vi "HFRR ADV v01.vi"() -> ()   [LabVIEW 2025] (continued)
          tunnel: w2263 -> [w2288 w2293]
          tunnel: [w2288 w2297] -> w2267
          tunnel: w2269 -> [w2287 w2292]
          tunnel: [w2287 w2295] -> w2275
          tunnel: w2265 -> [_ w2291]
          tunnel: [_ w2294] -> _
          frame False {
            # "DATA  WRITE LOOP"
          }
          frame True {
            n1901 = Concatenate Strings(w2291, "\r\n") -> (w2290:string)
            n1902 = VISA Write(VISA resource name=w2293, write buffer=w2290, error in (no error)=w2292) -> (VISA resource name out=w2297:refnum<visa-resource-name>, return count=w2294:u32, error out=w2296:errorcluster)
            n1903 = flat-sequence {
              tunnel: w2296 -> [w2299]
              tunnel: [w2299] -> w2295
              frame #0 {
                n1904 = local write "Due Write"("" ("Command")) -> ()
                n1905 = Wait (ms)(milliseconds to wait=u32 5) -> ()  [unwired: 1 out]
              }
            }
          }
        }
        "Port 2a" <- TRUE ("Port 2a")
      }
      frame Error {
        w2316 = u16 0 items=["None", "XON/XOFF", "RTS/CTS", "XON/XOFF & RTS/CTS", "DTR/DSR", "XON/XOFF & DTR/DSR"] ("flow control (0:none)  2")
        w2314 = u16 10 items=["1.0"=10, "1.5"=15, "2.0"=20] ("stop bits 2")
        w2312 = u16 0 items=["None", "Odd", "Even", "Mark", "Space"] ("parity 2")
        w2313 = u32 10000  # timeout (10sec)
        n1906 = VISA Clear(VISA resource name=w2308, error in (no error)=w2305) -> (VISA resource name out=w2307:refnum<visa-resource-name>, error out=w2306:errorcluster)
        n1907 = VISA Close(VISA resource name=w2307, error in (no error)=w2306) -> (error out=w2309:errorcluster)
        n1908 = call <vilib>:"Clear Errors.vi"("error in (no error)"=w2309) -> ()  [unwired: 5 in, 2 out]
        n1909 = local write "Port 2a"(FALSE ("Port 2a")) -> ()
        n1910 = local read "Com Port 2"() -> (w2302:refnum<visa-resource-name>)
        "visa due" <- w2302
        n1911 = call-poly "VISA Configure Serial Port"("VISA resource name"=w2302, "timeout (10sec)"=w2313, "baud rate (9600)"=u32 250000 ("baud rate  2"), "data bits (8)"=u16 8 ("data bits  2"), "parity (0:none)"=w2312, "stop bits (10: 1 bit)"=w2314, "flow control (0:none)"=w2316) -> ("VISA resource name out"=w2317:refnum<visa-resource-name>, "error out"=w2318:errorcluster)  [unwired: 7 in]
        n1912 = flat-sequence {
          tunnel: w2317 -> [w2320]
          tunnel: w2318 -> [w2319]
          tunnel: [w2320] -> w2310
          tunnel: [w2319] -> w2303
          frame #0 {
            n1913 = Wait (ms)(milliseconds to wait=u32 50) -> ()  [unwired: 1 out]
          }
        }
        "Residual Due" <- ""
      }
    }
    "error out 9" <- w2244
    n1914 = local read "Quit"() -> (w2246:bool)
    "Error Due" <- w2251
  }
  n1915 = local write "FRICVALZ"(0.0 ("FRICVALZ")) -> ()
  n1916 = property on="RUN" class="Bool (strict)"("Visible"=TRUE) -> ()  [unwired: 2 in, 2 out]
  n1917 = while {
    tunnel: [w2335] -> _
    tunnel: [w2322] -> w59
    i -> [w2335]
    stop <- w2322 stop-if-true
    n1918 = local read "conststatus"() -> (w2326:dbl)
    n1919 = local read "Main Tab"() -> (w2324:T4)
    n1920 = local read "EDIT"() -> (w2341:bool)
    n1921 = local read "Rate"() -> (w2340:dbl)
    n1922 = case shown="True" w2341 {
      tunnel: [FALSE TRUE] -> _
      frame False {
      }
      frame True {
      }
    }
    n1923 = Equal?(x=w2324, y=T28."About" ("Main Tab")) -> (x = y?=w2333:bool)
    n1924 = Equal?(x=w2326, y=0.0) -> (x = y?=w2327:bool)
    n1925 = Divide(x=1.0, y=w2340) -> (x/y=w2336:dbl)
    "Time 2" <- w2336
    n1926 = case shown="True" w2327 {
      frame False {
      }
      frame True {
        # "C:\\WinDucom\\calibrate WO 2391.dcf"
        n1927 = local write "Lan flag"(22) -> ()
        n1928 = local write "conststatus"(10.0 ("rpm value : 2")) -> ()
        n1929 = String To Path(string="C:\\LAB-IQ\\calibrate WO 2472.dcf") -> (path=w2347:path)
        n1930 = Open/Create/Replace File "Open File"(file path (use dialog)=w2347) -> (refnum out=w2345:refnum<file>)  [unwired: 5 in, 2 out]
        n1931 = for {
          N: 23 -> [_]
          tunnel: w2345 -> [w2356]
          i -> [w2350]
          (unwired) TRUE ("line mode (F)")
          n1932 = Read from Text File "Read File"(file (use dialog)=w2356) -> (text=w2355:string)  [unwired: 3 in, 3 out]
          n1933 = Match Pattern(string=w2355, regular expression="]") -> (after substring=w2353:string)  [unwired: 1 in, 3 out]
          n1934 = String Subset(string=w2355, offset (0)=5, length (rest)=10 ("length (rest)")) -> (substring=w2348:string)
          n1935 = Fract/Exp String To Number(string=w2348) -> (number=w2349:dbl)  [unwired: 3 in, 1 out]
          n1936 = Match Pattern(string=w2353, regular expression="-") -> (before substring=w2351:string)  [unwired: 1 in, 3 out]
          n1937 = case shown="10" w2350 {
            tunnel: w2349 -> [_ _ _ _ _ _ _ _ _ _ w2363 _ _ _ _ _ _ _ _ _ _ _ _ _]
            tunnel: w2351 -> [_ _ _ _ w2359 w2360 w2361 _ _ _ _ _ _ _ _ _ _ _ _ _ w2364 w2365 w2366 _]
            frame 0 {
            }
            frame 1 {
            }
            frame 2 {
            }
            frame 3 {
            }
            frame 4 {
              n1938 = local write "Com Port 1"(w2359) -> ()
            }
            frame 5 {
              n1939 = local write "Com Port 2"(w2360) -> ()
              n1940 = local write "visa due"(w2360) -> ()
            }
            frame 6 {
              n1941 = String To Path(string=w2361) -> (path=w2362:path)
              n1942 = local write "File Path"(w2362) -> ()
              "String" <- w2361
            }
            frame 7 {
            }
            frame 8 {
            }
            frame 9 {
            }
            frame 10 {
              n1943 = local write "Language Selection"(w2363) -> ()
            }
            frame 11 {
            }
            frame 12 {
            }
            frame 13 {
            }
            frame 14 {
            }
            frame 15 {
            }
            frame 16 {
            }
            frame 17 {
            }
            frame 18 {
            }
            frame 21 {
            }
            frame 22 {
              n1944 = local write "Com Port 3"(w2364) -> ()
            }
            frame 20 {
              n1945 = local write "Camera Port :"(w2365) -> ()
            }
            frame 19 {
              n1946 = local write "C3 :"(w2366) -> ()
            }
            frame 23, Default {
            }
          }
        }
      }
    }
    n1947 = Select(t=u32 2500 ("milliseconds to wait"), s=w2333, f=u32 500 ("milliseconds to wait")) -> (s? t:f=w2331:u32)
    n1948 = Multiply(x=w2336, y=w2331) -> (x*y=w2338:dbl)
    n1949 = call "Elapsed Time2"("Time Target (s)"=w2338, "Auto Reset"=TRUE) -> ("Time has Elapsed"=w2328:bool)  [unwired: 10 in, 7 out]
    n1950 = case shown="True" w2328 {
      frame False {
      }
      frame True {
        n1951 = stacked-sequence {
          frame #0 {
            # "DATA PROCESSING"
            # "115 mV/N"
            n1952 = local read "Sample Temperature 2"() -> (w2369:dbl)
            n1953 = local read "RH Numeric:"() -> (→"Humidity ( %RH )":dbl)
            n1954 = local read "FRICVALZ"() -> (w2386:dbl)
            n1955 = local read "Friction"() -> (w2372:dbl)
            n1956 = call <vilib>:"Mean PtByPt.vi"("x"=w2369, "sample length"=100) -> ("mean"=w2368:dbl)  [unwired: 2 in, 1 out]
            "TEMP 2" <- w2368
            "TEMP 3" <- w2368
            n1957 = Subtract(x=w2372, y=w2386) -> (x-y=w2381:dbl)
            "FF 2" <- w2381
            "FF 4" <- w2381
            n1958 = local read "Ambient Temperature"() -> (→"AIR TEMP":dbl)
            n1959 = local read "TEMP"() -> (w2385:dbl)
            n1960 = local write "FF 3"(w2381) -> ()
            n1961 = Compound Arithmetic op=OR("FRICVALZ 4", "FRICVALZ 3", "FRICVALZ 2") -> (w2377:bool)
            n1962 = case shown="True" w2377 {
              tunnel: w2372 -> [_ w2392]
              frame False {
              }
              frame True {
                w2391 = FALSE ("FRICVALZ")
                n1963 = local write "FRICVALZ 3"(w2391) -> ()
                n1964 = local write "FRICVALZ 2"(w2391) -> ()
                n1965 = local write "FRICVALZ 4"(w2391) -> ()
                "FRICVALZ" <- w2392
              }
            }
            n1966 = Not A Number/Path/Refnum?(number/path/refnum=w2385) -> (NaN/Path/Refnum?=w2384:bool)
            n1967 = Not A Number/Path/Refnum?(number/path/refnum=w2381) -> (NaN/Path/Refnum?=w2383:bool)
            n1968 = Divide(x=w2381, y=1.96) -> (x/y=w2378:dbl)
            n1969 = Compound Arithmetic op=OR(w2384, w2383) -> (w2382:bool)
            n1970 = Not A Number/Path/Refnum?(number/path/refnum=w2378) -> (NaN/Path/Refnum?=w2379:bool)
            n1971 = case shown="True" w2382 {
              frame False {
              }
              frame True {
                n1972 = local write "TEMP"(0.0 ("TEMP")) -> ()
                n1973 = local write "FF 2"(0.0 ("FF 2")) -> ()
                n1974 = local write "reinit"(TRUE ("reinit")) -> ()
              }
            }
            n1975 = local write "TEMP"(w2368) -> ()
            n1976 = Select(t=0.0, s=w2379, f=w2378) -> (s? t:f=w2371:dbl)
            "COF 2" <- w2371
            n1977 = local write "COF 3"(w2371) -> ()
          }
        }
      }
    }
    n1978 = Wait (ms)(milliseconds to wait=u32 50) -> ()  [unwired: 1 out]
    n1979 = local read "Quit"() -> (w2322:bool)
    "Rate" <- 2500.0 ("No of Samples")
  }
  n1980 = while {
    tunnel: [w2412] -> _
    tunnel: [w2395] -> w61
    tunnel: w6 -> [_]
    i -> [w2412]
    stop <- w2395 stop-if-true
    # "C:\\LAB-IQ-NXT\\Scar View.exe"
    n1981 = local read "OK Button 16"() -> (w2402:bool)
    n1982 = local read "Main Tab"() -> (w2396:T4)
    n1983 = local read "service 3"() -> (w2397:bool)
    n1984 = local read "OPEN 6"() -> (w2399:bool)
    n1985 = local read "EDIT 2"() -> (w2401:bool)
    n1986 = flat-sequence {
      frame #0 {
        n1987 = stacked-sequence {
          frame #0 {
            n1988 = local read "EDIT"() -> (w2890:bool)
            n1989 = case shown="False" w2890 {
              tunnel: [u8 2 ("Disabled") u8 0 ("Disabled")] -> _
              frame False {
                w2892 = FALSE
                n1990 = local write "Password"("") -> ()
                n1991 = local write "x = y?"(w2892) -> ()
                n1992 = property on="Password" class="Str"("Visible"=w2892) -> ()  [unwired: 2 in, 2 out]
              }
              frame True {
                n1993 = property on="Password" class="Str"("Visible"=TRUE) -> ()  [unwired: 2 in, 2 out]
              }
            }
            "dipl pwd" <- "@143$\n" ("dipl pwd")
          }
          frame #1 {
          }
          frame #2 {
          }
          frame #3 {
          }
          frame #4 {
            n1994 = String To Byte Array(string="Password") -> (unsigned byte array=w2903:u8[])
            n1995 = Search 1D Array(1D array=w2903, element=u8 10) -> (index of element=w2901:i32)  [unwired: 1 in]
            n1996 = Index Array(array=w2903, index=w2901) -> (element=w2902:u8)
            n1997 = Equal?(x=w2902, y=10) -> (x = y?=w2898:bool)
            n1998 = case shown="True" w2898 {
              frame False {
              }
              frame True {
                # "password"
                # "password"
                n1999 = local read "Password"() -> (w2915:string)
                n2000 = String To Byte Array(string=w2915) -> (unsigned byte array=w2918:u8[])
                n2001 = String To Byte Array(string="@143$\n") -> (unsigned byte array=w2905:u8[])
                n2002 = Array Size(array=w2918) -> (size(s)=w2914:i32)
                n2003 = Array Size(array=w2905) -> (size(s)=w2910:i32)
                n2004 = for {
                  N: w2914 -> [_]
                  tunnel: w2918 -> [w2931]
                  tunnel: [w2929] -> w2919 mode=indexing
                  tunnel: w2914 -> [w2926]
                  i -> [w2927]
                  n2005 = Decrement(x=w2926) -> (x-1=w2925:i32)
                  n2006 = Index Array(array=w2931, index=w2927) -> (element=w2930:u8)
                  n2007 = Equal?(x=w2927, y=w2925) -> (x = y?=w2924:bool)
                  n2008 = Number To Decimal String(number=w2930) -> (decimal integer string=w2928:string)  [unwired: 1 in]
                  n2009 = Select(t="", s=w2924, f="\r") -> (s? t:f=w2921:string)
                  n2010 = Concatenate Strings(w2928, w2921) -> (w2929:string)
                }
                n2011 = for {
                  N: w2910 -> [_]
                  tunnel: w2905 -> [w2942]
                  tunnel: [w2940] -> w2908 mode=indexing
                  tunnel: w2910 -> [w2937]
                  i -> [w2938]
                  n2012 = Decrement(x=w2937) -> (x-1=w2936:i32)
                  n2013 = Index Array(array=w2942, index=w2938) -> (element=w2941:u8)
                  n2014 = Equal?(x=w2938, y=w2936) -> (x = y?=w2935:bool)
                  n2015 = Number To Decimal String(number=w2941) -> (decimal integer string=w2939:string)  [unwired: 1 in]
                  n2016 = Select(t="", s=w2935, f="\r") -> (s? t:f=w2932:string)
                  n2017 = Concatenate Strings(w2939, w2932) -> (w2940:string)
                }
                n2018 = local read "file path"() -> (w2904:path)
                n2019 = call <vilib>:"Read Characters From File.vi"("file path (dialog if empty)"=w2904) -> ("character string"=w2917:string)  [unwired: 5 in, 3 out]
                "string" <- w2917
                n2020 = flat-sequence {
                  tunnel: [w2920] -> _
                  frame #0 {
                    w2920 = ""
                    n2021 = local write "Password"(w2920) -> ()
                  }
                }
                n2022 = Concatenate Strings(w2908) -> (w2909:string)
                n2023 = Concatenate Strings(w2917) -> (w2916:string)
                n2024 = Concatenate Strings(w2919) -> (w2912:string)
                n2025 = Equal?(x=w2912, y=w2916) -> (x = y?=w2907:bool)
                n2026 = Equal?(x=w2912, y=w2909) -> (x = y?=w2913:bool)
                n2027 = Or(x=w2907, y=w2913) -> (x .or. y?=→"x = y?":bool)
              }
            }
          }
        }
        n2028 = local read "x = y?"() -> (w2888:bool)
        n2029 = And(x="EDIT", y=w2888) -> (x .and. y?=w2886:bool)
        n2030 = case shown="True" w2886 {
          tunnel: [u8 2 ("Disabled") u8 0 ("Disabled")] -> w2885
          tunnel: [w3092 TRUE ("Visible")] -> w2884
          frame False {
            w3092 = FALSE ("Visible")
            n2031 = local write "EDIT 2"(w3092) -> ()
          }
          frame True {
          }
        }
        n2032 = case shown="True" "SAVE" {
          frame False {
          }
          frame True {
            n2033 = stacked-sequence {
              seq-local: [w2947 _ _] -> [_ w3088 _]
              frame #0 {
                w2943 = 0.0 ("number")
                w2944 = 0.0 ("number")
                (unwired) i16 5 ("precision (6)")
                # "[CH1]    - FF\n[CH2]   - TEMPERATURE\n[CH3]    - Humidity\n[CH4]    - AIR TEMP\n[CH5]\\- Visa Uno\n[CH6] \\- Visa Due\n[CH7]  \\- file path\n[CH8]   - Displacement Gain\n[CHA]   - Stroke Gain\n[CHB]   - Stroke PID Gain\n[CHC]   -Language Selection\n[CHD]   -Power +\n[CHE]   -Power_\n[CHF]   -Heater\n[CHG]   -Humidity Wet\n[CHH]   -Humidity Dry\n[CHI]   -Integral Time"
                n2034 = local read "Language Selection"() -> (w2990:enum16{"English", "Russian"})
                n2035 = Path To String(path="File Path") -> (string=w3006:string)
                n2036 = Number To Fractional String(number=w2943, width (-)=i16 10 ("precision (6)"), precision (6)=i16 5) -> (F-format string=w2997:string)  [unwired: 1 in]
                n2037 = Number To Fractional String(number=w2990, width (-)=i16 10 ("precision (6)"), precision (6)=i16 5) -> (F-format string=w2986:string)  [unwired: 1 in]
                n2038 = Number To Fractional String(number=w2944, width (-)=i16 10 ("precision (6)"), precision (6)=i16 5) -> (F-format string=w2980:string)  [unwired: 1 in]
                n2039 = Number To Fractional String(number=w2944, width (-)=i16 10 ("precision (6)"), precision (6)=i16 5) -> (F-format string=w2977:string)  [unwired: 1 in]
                n2040 = Number To Fractional String(number=w2944, width (-)=i16 10 ("precision (6)"), precision (6)=i16 5) -> (F-format string=w2972:string)  [unwired: 1 in]
                n2041 = Number To Fractional String(number=w2944, width (-)=i16 10 ("precision (6)"), precision (6)=i16 5) -> (F-format string=w2969:string)  [unwired: 1 in]
                n2042 = Number To Fractional String(number=w2944, width (-)=i16 10 ("precision (6)"), precision (6)=i16 5) -> (F-format string=w2964:string)  [unwired: 1 in]
                n2043 = local read "Com Port 1"() -> (w2946:refnum<visa-resource-name>)
                n2044 = local read "Com Port 2"() -> (w2945:refnum<visa-resource-name>)
                n2045 = Concatenate Strings(w3006, "\\" ("string")) -> (w3005:string)
                n2046 = Number To Fractional String(number=w2943, width (-)=i16 10 ("precision (6)"), precision (6)=i16 5) -> (F-format string=w3038:string)  [unwired: 1 in]
                n2047 = Number To Fractional String(number=w2943, width (-)=i16 10 ("precision (6)"), precision (6)=i16 5) -> (F-format string=w3037:string)  [unwired: 1 in]
                n2048 = Number To Fractional String(number=w2943, width (-)=i16 10 ("precision (6)"), precision (6)=i16 5) -> (F-format string=w3031:string)  [unwired: 1 in]
                n2049 = Number To Fractional String(number=w2943, width (-)=i16 10 ("precision (6)"), precision (6)=i16 5) -> (F-format string=w3025:string)  [unwired: 1 in]
                n2050 = Number To Fractional String(number=w2943, width (-)=i16 10 ("precision (6)"), precision (6)=i16 5) -> (F-format string=w2998:string)  [unwired: 1 in]
                n2051 = Concatenate Strings("[CHA]" ("string"), w2997, "- Stroke Gain" ("string"), "\r") -> (w2991:string)
                n2052 = Concatenate Strings("[CHC]" ("string"), w2986, "-Language Selection" ("string"), "\r") -> (w2983:string)
                n2053 = Concatenate Strings("[CHD]" ("string"), w2980, "-Power +" ("string"), "\r") -> (w2962:string)
                n2054 = Concatenate Strings("[CHG]" ("string"), w2969, "-Humidity Wet" ("string"), "\r") -> (w2959:string)
                n2055 = Concatenate Strings("[CHH]" ("string"), w2964, "-Humidity Dry" ("string"), "\r") -> (w2958:string)
                n2056 = Concatenate Strings("[CH1]" ("string"), w3038, " - FF" ("string"), "\r") -> (w3036:string)
                n2057 = Concatenate Strings("[CH2]" ("string"), w3037, " - TEMPERATURE" ("string"), "\r") -> (w3035:string)
                n2058 = Concatenate Strings("[CH3]" ("string"), w3031, " - Humidity" ("string"), "\r") -> (w3028:string)
                n2059 = Concatenate Strings("[CH4]" ("string"), w3025, " - AIR TEMP" ("string"), "\r") -> (w3021:string)
                n2060 = Concatenate Strings("[CH5]" ("string"), w2946, "- Visa Uno" ("string"), "\r") -> (w3014:string)
                n2061 = Concatenate Strings("[CH6]" ("string"), w2945, "- Visa Due" ("string"), "\r") -> (w3009:string)
                n2062 = Concatenate Strings("[CH7]" ("string"), w3005, "- file path" ("string"), "\r") -> (w3008:string)
                n2063 = Concatenate Strings("[CH8]" ("string"), w2998, "- Displacement Gain" ("string"), "\r") -> (w3001:string)
                n2064 = Concatenate Strings("[CHE]" ("string"), w2977, "-Power_" ("string"), "\r") -> (w2961:string)
                n2065 = Concatenate Strings("[CHF]" ("string"), w2972, "-Heater" ("string"), "\r") -> (w2960:string)
                n2066 = Concatenate Strings(w3036, w3035, w3028, w3021, w3014, w3009, w3008, w3001, w2991, w2983, w2962, w2961, w2960, w2959, w2958) -> (w2947:string)
                "gain" <- w2947
              }
              frame #1 {
                w3049 = 0.0 ("number")
                n2067 = local read "Camera Port :"() -> (w3052:string)
                n2068 = local read "C3 :"() -> (w3060:refnum<visa-resource-name>)
                n2069 = local read "Com Port 3"() -> (w3061:refnum<visa-resource-name>)
                n2070 = Concatenate Strings("[CH8]" ("string"), w3052, "- Visa Camera" ("string"), "\r") -> (w3051:string)
                n2071 = Concatenate Strings("[CH7]" ("string"), w3060, "- Visa Humidity" ("string"), "\r") -> (w3056:string)
                n2072 = Number To Fractional String(number=w3049, width (-)=i16 10 ("precision (6)"), precision (6)=i16 5) -> (F-format string=w3076:string)  [unwired: 1 in]
                n2073 = Concatenate Strings("[CHL]" ("string"), w3061, "- Visa humid" ("string"), "\r") -> (w3064:string)
                n2074 = Number To Fractional String(number=w3049, width (-)=i16 10 ("precision (6)"), precision (6)=i16 5) -> (F-format string=w3083:string)  [unwired: 1 in]
                n2075 = Concatenate Strings("[CHK]" ("string"), w3076, "-TEMP INTERCEPT" ("string"), "\r") -> (w3072:string)
                n2076 = Concatenate Strings("[SNO]" ("string"), "" ("string"), "-" ("string"), "\r") -> (w3069:string)
                n2077 = Concatenate Strings("[CHJ]" ("string"), w3083, "-AIR TEMP INTERCEPT" ("string"), "\r") -> (w3073:string)
                n2078 = String To Path(string="C:\\LAB-IQ\\calibrate WO 2472.dcf") -> (path=w3062:path)
                n2079 = Concatenate Strings(w3088, w3073, w3072, w3069, w3064, w3056, w3051) -> (w3087:string)
                n2080 = call <vilib>:"Write Characters To File.vi"("append to file? (new file:F)"=FALSE, "character string"=w3087, "file path (dialog if empty)"=w3062) -> ()  [unwired: 2 in, 1 out]
              }
              frame #2 {
                n2081 = local write "Lan flag"(0.0 ("Lan flag")) -> ()
                n2082 = local write "conststatus"(0.0 ("rpm value : 2")) -> ()
                n2083 = local write "SAVE"(FALSE ("OK Button 14")) -> ()
              }
            }
          }
        }
        n2084 = property on="EDIT 2" class="Bool (strict)"("Visible"=w2884) -> ()  [unwired: 2 in, 2 out]
        n2085 = property on="SAVE" class="Bool (strict)"("Visible"=w2884) -> ()  [unwired: 2 in, 2 out]
        n2086 = property on="visa due" class="CmbBox"("Disabled"=w2885) -> ()  [unwired: 2 in, 2 out]
        n2087 = property on="File Path" class="Path"("Disabled"=w2885) -> ()  [unwired: 2 in, 2 out]
        n2088 = property on="Language Selection" class="Enum (strict)"("Visible"=w2884) -> ()  [unwired: 2 in, 2 out]
        n2089 = property on="SPEED OUT:" class="DigNum (strict)"("Disabled"=w2885) -> ()  [unwired: 2 in, 2 out]
      }
    }
    n2090 = local read "RUN"() -> (w2411:bool)
    n2091 = local read "RUN"() -> (w2409:bool)
    n2092 = case shown="True" "EDIT 3" {
      frame False {
      }
      frame True {
        n2093 = local write "EDIT 3"(FALSE ("EDIT 3")) -> ()
        n2094 = local write "Main Tab"(T4."About" ("Main Tab")) -> ()
      }
    }
    n2095 = case shown="False" w2411 {
      frame False {
        n2096 = local read "stopT"() -> (w3099:bool)
        n2097 = case shown="True" w3099 {
          frame False {
          }
          frame True {
            n2098 = local write "stopT"(FALSE) -> ()
          }
        }
      }
      frame True {
        "stopT" <- TRUE
      }
    }
    n2099 = case shown="False" w2409 {
      frame False {
      }
      frame True {
      }
    }
    n2100 = case shown="True" w2401 {
      frame False {
        n2101 = property on="Password 2" class="Str"("Visible"=FALSE) -> ()  [unwired: 2 in, 2 out]
        n2102 = local write "Password 2"("" ("Password")) -> ()
      }
      frame True {
        n2103 = property on="Password 2" class="Str"("Visible"=TRUE) -> ()  [unwired: 2 in, 2 out]
        n2104 = Equal?(x="Password 2", y="HFRR1234") -> (x = y?=w2424:bool)
        n2105 = case shown="True" w2424 {
          tunnel: "Password 2" -> [w2427 _]
          frame False {
            n2106 = String Length(string=w2427) -> (length=w2428:i32)
            n2107 = Greater Than 0?(x=w2428) -> (x > 0?=w2426:bool)
            n2108 = case shown="False" w2426 {
              frame False {
                n2109 = property on="Password 2" class="Str"("Caption.Text"="Password (Advance Setting)") -> ()  [unwired: 2 in, 2 out]
              }
              frame True {
                n2110 = property on="Password 2" class="Str"("Caption.Text"="Incorrect Password!") -> ()  [unwired: 2 in, 2 out]
              }
            }
          }
          frame True {
            n2111 = local write "EDIT 2"(FALSE ("EDIT 2")) -> ()
            n2112 = local write "Password 2"("" ("Password")) -> ()
            n2113 = local write "Main Tab"(T4."Advance" ("Main Tab")) -> ()
            n2114 = local write "Main Dashboard Buttons"(T1."Advance" ("Main Dashboard Buttons")) -> ()
          }
        }
      }
    }
    n2115 = case shown="True" "Prog Uno" {
      frame False {
      }
      frame True {
        n2116 = stacked-sequence {
          frame #0 {
            n2117 = Delete(path (use dialog)=path "C:/LAB-IQ-NXT/UNOCOMPILE.bat" ("working directory")) -> ()  [unwired: 4 in, 3 out]
          }
          frame #1 {
            n2118 = local read "Com Port 1"() -> (w2866:refnum<visa-resource-name>)
            n2119 = Concatenate Strings("cmd.exe /c \"mode " ("command line"), w2866, ":1200,n,8,1\"\n" ("command line")) -> (w2871:string)
            n2120 = Concatenate Strings(w2871, "CD\\\nCD WinDucom\navrdude -C avrdude.conf -v -patmega328p -carduino -P" ("command line"), w2866, " -b115200 -D -Uflash:w:UNO_V20.hex:i\n" ("command line"), "\r") -> (w2873:string)
            "STR" <- w2873
            n2121 = call <vilib>:"Write Characters To File.vi"("append to file? (new file:F)"=FALSE, "character string"=w2873, "file path (dialog if empty)"=path "C:/LAB-IQ/UNOCOMPILE.bat" ("working directory")) -> ()  [unwired: 2 in, 1 out]
          }
          frame #2 {
            n2122 = disable-structure shown="Disabled" {
              frame Disabled {
                w2877 = "cmd.exe  /c \"C:\\LAB-IQ-NXT\\UNOCOMPILE.bat\"" ("string")
                n2123 = local write "Prog Uno"(FALSE ("run minimized? (F)")) -> ()
                n2124 = call <vilib>:"System Exec.vi"("expected output size  (4096)"=u32 65535, "run minimized? (F)"=FALSE, "wait until completion? (T)"=TRUE ("run minimized? (F)"), "working directory"=path "C:/LAB-IQ-NXT", "standard input"=w2877, "command line"=w2877) -> ("error out"=w2876:errorcluster, "standard output"=→"String 42":string)  [unwired: 2 in, 2 out]
                "error out 3" <- w2876
                n2125 = flat-sequence {
                  tunnel: w2876 -> [_]
                  frame #0 {
                  }
                }
              }
              frame Enabled {
              }
            }
          }
        }
      }
    }
    n2126 = case shown="\"ISO 12156\"" "TEST STANDARD" {
      frame "ASTM D6079", Default {
        w2846 = 50.0 ("Hz")
        w2847 = 53.0 ("Set Rh")
        w2849 = 1.0 ("Set Strk")
        w2848 = 60.0 ("Set Temp")
        # "astm hide"
        n2127 = local write "NORMAL LOAD"(200.0 ("NORMAL LOAD")) -> ()
        n2128 = local write "Set Strk"(w2849) -> ()
        n2129 = local write "Set Hz"(w2846) -> ()
        n2130 = local write "Set Temp"(w2848) -> ()
        n2131 = local write "Set Rh"(w2847) -> ()
        n2132 = local write "test time"(75.0 ("test time")) -> ()
        n2133 = local write "Set Stroke:"(w2849) -> ()
        n2134 = local write "Set Humidity:"(w2847) -> ()
        n2135 = local write "Set Frequency:"(w2846) -> ()
        n2136 = local write "Set Temperature:"(w2848) -> ()
        "Test Standard" <- "ASTM D6079" ("Test Standard 2")
      }
      frame "ISO 12156" {
        n2137 = local write "Set Strk"(1.0 ("Set Strk")) -> ()
        n2138 = local write "NORMAL LOAD"(200.0 ("NORMAL LOAD")) -> ()
        n2139 = local write "Set Temp"(60.0 ("Set Temp")) -> ()
        n2140 = local write "test time"(75.0 ("test time")) -> ()
        n2141 = local write "Set Hz"(50.0 ("Hz")) -> ()
        n2142 = local write "Set Rh"(53.0 ("Set Rh")) -> ()
      }
      frame "CEC F-096-A-06" {
        n2143 = local write "Set Strk"(1.0 ("Set Strk")) -> ()
        n2144 = local write "NORMAL LOAD"(200.0 ("NORMAL LOAD")) -> ()
        n2145 = local write "Set Temp"(60.0 ("Set Temp")) -> ()
        n2146 = local write "test time"(75.0 ("test time")) -> ()
        n2147 = local write "Set Hz"(50.0 ("Hz")) -> ()
        n2148 = local write "Set Rh"(53.0 ("Set Rh")) -> ()
      }
      frame "Custom" {
      }
    }
    n2149 = Or(x=w2399, y=w2397) -> (x .or. y?=w2398:bool)
    n2150 = case shown="\"About\"" w2396 {
      tunnel: [T28."Acquire" ("Main Tab") T28."Compare Files" ("Main Tab") T28."About" ("Main Tab")] -> w2407
      frame "Acquire", Default {
      }
      frame "Compare Files" {
      }
      frame "About" {
      }
    }
    n2151 = Or(x=w2402, y="OPEN") -> (x .or. y?=w2403:bool)
    n2152 = case shown="True" w2403 {
      tunnel: w2402 -> [_ w2435]
      frame False {
      }
      frame True {
        n2153 = stacked-sequence {
          tunnel: w2435 -> [_ w2502 _ _]
          frame #0 {
            w2451 = "  " ("String 6")
            n2154 = local write "OPEN"(FALSE ("open")) -> ()
            n2155 = local read "string1 2"() -> (w2439:string)
            n2156 = local read "string1 3"() -> (w2438:string)
            n2157 = local read "string1 4"() -> (w2437:string)
            n2158 = property on="OPEN" class="Bool (strict)"("Visible"=FALSE) -> ()  [unwired: 2 in, 2 out]
            n2159 = local write "String 6"(w2451) -> ()
            n2160 = local write "String 7"(w2451) -> ()
            n2161 = local write "String 8"(w2451) -> ()
            n2162 = local write "String 12"(w2451) -> ()
            n2163 = local read "OK Button 16"() -> (w2436:bool)
            n2164 = String To Path(string=w2439) -> (path=w2447:path)
            n2165 = String To Path(string=w2438) -> (path=w2446:path)
            n2166 = String To Path(string=w2437) -> (path=w2445:path)
            n2167 = case shown="True" w2436 {
              tunnel: [w2452 w2453] -> w2440
              frame False {
                n2168 = local read "string1"() -> (w2452:string)
              }
              frame True {
                n2169 = local read "String Indicator 4"() -> (w2453:string)
              }
            }
            n2170 = Open/Create/Replace File "Open File"(file path (use dialog)=w2447) -> (refnum out=w2443:refnum<file>)  [unwired: 5 in, 2 out]
            n2171 = Open/Create/Replace File "Open File"(file path (use dialog)=w2446) -> (refnum out=w2442:refnum<file>)  [unwired: 5 in, 2 out]
            n2172 = Open/Create/Replace File "Open File"(file path (use dialog)=w2445) -> (refnum out=w2441:refnum<file>)  [unwired: 5 in, 2 out]
            n2173 = while {
              tunnel: w2443 -> [w2465]
              i -> [w2461]
              stop <- w2460 continue-if-true
              (unwired) TRUE ("line mode (F)")
              n2174 = Read from Text File "Read File"(file (use dialog)=w2465) -> (text=w2462:string)  [unwired: 3 in, 3 out]
              n2175 = local write "Numeric 11"(w2461) -> ()
              n2176 = String Length(string=w2462) -> (length=w2464:i32)
              n2177 = Greater?(x=w2464, y=1) -> (0:w2460:bool)
            }
            n2178 = while {
              tunnel: w2442 -> [w2471]
              i -> [w2467]
              stop <- w2466 continue-if-true
              (unwired) TRUE ("line mode (F)")
              n2179 = Read from Text File "Read File"(file (use dialog)=w2471) -> (text=w2468:string)  [unwired: 3 in, 3 out]
              n2180 = local write "Numeric 12"(w2467) -> ()
              n2181 = String Length(string=w2468) -> (length=w2470:i32)
              n2182 = Greater?(x=w2470, y=1) -> (0:w2466:bool)
            }
            n2183 = while {
              tunnel: w2441 -> [w2477]
              i -> [w2473]
              stop <- w2472 continue-if-true
              (unwired) TRUE ("line mode (F)")
              n2184 = Read from Text File "Read File"(file (use dialog)=w2477) -> (text=w2474:string)  [unwired: 3 in, 3 out]
              n2185 = local write "Numeric 13"(w2473) -> ()
              n2186 = String Length(string=w2474) -> (length=w2476:i32)
              n2187 = Greater?(x=w2476, y=1) -> (0:w2472:bool)
            }
            n2188 = String To Path(string=w2440) -> (path=w2448:path)
            n2189 = Open/Create/Replace File "Open File"(file path (use dialog)=w2448) -> (refnum out=w2444:refnum<file>)  [unwired: 5 in, 2 out]
            n2190 = while {
              tunnel: w2444 -> [w2459]
              i -> [w2455]
              stop <- w2454 continue-if-true
              (unwired) TRUE ("line mode (F)")
              n2191 = Read from Text File "Read File"(file (use dialog)=w2459) -> (text=w2456:string)  [unwired: 3 in, 3 out]
              n2192 = local write "Numeric 8"(w2455) -> ()
              n2193 = String Length(string=w2456) -> (length=w2458:i32)
              n2194 = Greater?(x=w2458, y=1) -> (0:w2454:bool)
            }
          }
          frame #1 {
            w2629 = FALSE ("ACTUAL   MERGE")
            # "Sample Temp"
            # "ECR"
            # "COF"
            # "Time\nCOF\nFF\nTemp"
            n2195 = case shown="True" w2502 {
              tunnel: [w2649 w2650] -> w2503
              frame False {
                n2196 = local read "string1"() -> (w2649:string)
              }
              frame True {
                n2197 = local read "String Indicator 4"() -> (w2650:string)
              }
            }
            n2198 = local read "string1 3"() -> (w2547:string)
            n2199 = String To Path(string=w2503) -> (path=w2634:path)
            n2200 = String To Path(string=w2547) -> (path=w2645:path)
            n2201 = local read "Numeric 12"() -> (w2631:i32)
            n2202 = local read "Numeric 8"() -> (w2633:i32)
            n2203 = local read "string1 2"() -> (w2548:string)
            n2204 = local read "string1 4"() -> (w2546:string)
            n2205 = Open/Create/Replace File "Open File"(file path (use dialog)=w2634) -> (refnum out=w2648:refnum<file>, error out=w2647:errorcluster)  [unwired: 5 in, 1 out]
            n2206 = Open/Create/Replace File "Open File"(file path (use dialog)=w2645) -> (refnum out=w2641:refnum<file>, error out=w2642:errorcluster)  [unwired: 5 in, 1 out]
            n2207 = for {
              N: w2633 -> [_]
              tunnel: w2648 -> [w2796]
              tunnel: w2647 -> [w2795]
              tunnel: [w2785] -> w2560 mode=indexing
              tunnel: [w2783] -> w2617 mode=indexing
              tunnel: [w2784] -> w2612 mode=indexing
              tunnel: w2629 -> [_]
              tunnel: [w2777] -> w2614 mode=indexing
              tunnel: [w2773] -> w2583 mode=indexing
              tunnel: [w2769] -> w2558 mode=indexing
              tunnel: [w2765] -> w2539 mode=indexing
              tunnel: [w2760] -> w2499 mode=indexing
              (unwired) TRUE ("line mode (F)")
              # "freq"
              # "Stroke"
              # "Time"
              # "CoF"
              # "Humidity"
              # "Temp"
              # "Air Temp"
              # "ECR"
              n2208 = Read from Text File "Read File"(file (use dialog)=w2796, error in=w2795) -> (text=w2761:string)  [unwired: 2 in, 3 out]
              n2209 = local write "String 6"(w2761) -> ()
              n2210 = String Subset(string=w2761, offset (0)=0, length (rest)=14 ("length (rest)")) -> (substring=w2789:string)
              n2211 = String Subset(string=w2761, offset (0)=35, length (rest)=9 ("length (rest)")) -> (substring=w2786:string)
              n2212 = String Subset(string=w2761, offset (0)=15, length (rest)=9 ("length (rest)")) -> (substring=w2792:string)
              n2213 = Fract/Exp String To Number(string=w2789) -> (number=w2785:dbl)  [unwired: 3 in, 1 out]
              n2214 = Fract/Exp String To Number(string=w2786) -> (number=w2784:dbl)  [unwired: 3 in, 1 out]
              n2215 = Fract/Exp String To Number(string=w2792) -> (number=w2783:dbl)  [unwired: 3 in, 1 out]
              n2216 = String Subset(string=w2761, offset (0)=85, length (rest)=9 ("length (rest)")) -> (substring=w2762:string)
              n2217 = String Subset(string=w2761, offset (0)=25, length (rest)=9 ("length (rest)")) -> (substring=w2768:string)
              n2218 = String Subset(string=w2761, offset (0)=55, length (rest)=9 ("length (rest)")) -> (substring=w2770:string)
              n2219 = String Subset(string=w2761, offset (0)=45, length (rest)=9 ("length (rest)")) -> (substring=w2776:string)
              n2220 = String Subset(string=w2761, offset (0)=65, length (rest)=9 ("length (rest)")) -> (substring=w2782:string)
              n2221 = Fract/Exp String To Number(string=w2768) -> (number=w2765:dbl)  [unwired: 3 in, 1 out]
              n2222 = Fract/Exp String To Number(string=w2762) -> (number=w2760:dbl)  [unwired: 3 in, 1 out]
              n2223 = Fract/Exp String To Number(string=w2770) -> (number=w2769:dbl)  [unwired: 3 in, 1 out]
              n2224 = Fract/Exp String To Number(string=w2776) -> (number=w2773:dbl)  [unwired: 3 in, 1 out]
              n2225 = Fract/Exp String To Number(string=w2782) -> (number=w2779:dbl)  [unwired: 3 in, 1 out]
              n2226 = Add(x=w2779, y=0.0) -> (x+y=w2777:dbl)
            }
            n2227 = for {
              N: w2631 -> [_]
              tunnel: w2642 -> [w2722]
              tunnel: w2641 -> [w2721]
              tunnel: [w2711] -> w2600 mode=indexing
              tunnel: [w2709] -> w2598 mode=indexing
              tunnel: [w2710] -> w2594 mode=indexing
              tunnel: w2629 -> [_]
              tunnel: [w2703] -> w2596 mode=indexing
              tunnel: [w2699] -> w2578 mode=indexing
              tunnel: [w2695] -> w2554 mode=indexing
              tunnel: [w2692] -> w2535 mode=indexing
              tunnel: [w2688] -> w2494 mode=indexing
              (unwired) 9 ("length (rest)")
              (unwired) 9 ("length (rest)")
              (unwired) TRUE ("line mode (F)")
              n2228 = Read from Text File "Read File"(file (use dialog)=w2721, error in=w2722) -> (text=w2689:string)  [unwired: 2 in, 3 out]
              n2229 = local write "String 8"(w2689) -> ()
              n2230 = String Subset(string=w2689, offset (0)=85) -> (substring=w2691:string)  [unwired: 1 in]
              n2231 = String Subset(string=w2689, offset (0)=35, length (rest)=9 ("length (rest)")) -> (substring=w2712:string)
              n2232 = String Subset(string=w2689, offset (0)=55, length (rest)=9 ("length (rest)")) -> (substring=w2697:string)
              n2233 = String Subset(string=w2689, offset (0)=25) -> (substring=w2693:string)  [unwired: 1 in]
              n2234 = String Subset(string=w2689, offset (0)=15, length (rest)=9 ("length (rest)")) -> (substring=w2718:string)
              n2235 = String Subset(string=w2689, offset (0)=0, length (rest)=14 ("length (rest)")) -> (substring=w2715:string)
              n2236 = String Subset(string=w2689, offset (0)=45, length (rest)=9 ("length (rest)")) -> (substring=w2702:string)
              n2237 = String Subset(string=w2689, offset (0)=65, length (rest)=9 ("length (rest)")) -> (substring=w2708:string)
              n2238 = Fract/Exp String To Number(string=w2691) -> (number=w2688:dbl)  [unwired: 3 in, 1 out]
              n2239 = Fract/Exp String To Number(string=w2712) -> (number=w2710:dbl)  [unwired: 3 in, 1 out]
              n2240 = Fract/Exp String To Number(string=w2697) -> (number=w2695:dbl)  [unwired: 3 in, 1 out]
              n2241 = Fract/Exp String To Number(string=w2693) -> (number=w2692:dbl)  [unwired: 3 in, 1 out]
              n2242 = Fract/Exp String To Number(string=w2718) -> (number=w2709:dbl)  [unwired: 3 in, 1 out]
              n2243 = Fract/Exp String To Number(string=w2715) -> (number=w2711:dbl)  [unwired: 3 in, 1 out]
              n2244 = Fract/Exp String To Number(string=w2702) -> (number=w2699:dbl)  [unwired: 3 in, 1 out]
              n2245 = Fract/Exp String To Number(string=w2708) -> (number=w2705:dbl)  [unwired: 3 in, 1 out]
              n2246 = Add(x=w2705, y=0.0) -> (x+y=w2703:dbl)
            }
            n2247 = String To Path(string=w2548) -> (path=w2646:path)
            n2248 = String To Path(string=w2546) -> (path=w2640:path)
            n2249 = local read "Numeric 11"() -> (w2630:i32)
            n2250 = local read "Numeric 13"() -> (w2632:i32)
            n2251 = Open/Create/Replace File "Open File"(file path (use dialog)=w2646) -> (refnum out=w2644:refnum<file>, error out=w2643:errorcluster)  [unwired: 5 in, 1 out]
            n2252 = Open/Create/Replace File "Open File"(file path (use dialog)=w2640) -> (refnum out=w2639:refnum<file>, error out=w2638:errorcluster)  [unwired: 5 in, 1 out]
            n2253 = for {
              N: w2630 -> [_]
              tunnel: w2644 -> [w2759]
              tunnel: w2643 -> [w2758]
              tunnel: [w2748] -> w2610 mode=indexing
              tunnel: [w2746] -> w2608 mode=indexing
              tunnel: [w2747] -> w2603 mode=indexing
              tunnel: w2629 -> [_]
              tunnel: [w2740] -> w2605 mode=indexing
              tunnel: [w2736] -> w2581 mode=indexing
              tunnel: [w2732] -> w2556 mode=indexing
              tunnel: [w2728] -> w2537 mode=indexing
              tunnel: [w2723] -> w2495 mode=indexing
              (unwired) TRUE ("line mode (F)")
              n2254 = Read from Text File "Read File"(file (use dialog)=w2759, error in=w2758) -> (text=w2724:string)  [unwired: 2 in, 3 out]
              n2255 = local write "String 7"(w2724) -> ()
              n2256 = String Subset(string=w2724, offset (0)=85, length (rest)=9 ("length (rest)")) -> (substring=w2727:string)
              n2257 = String Subset(string=w2724, offset (0)=35, length (rest)=9 ("length (rest)")) -> (substring=w2749:string)
              n2258 = String Subset(string=w2724, offset (0)=55, length (rest)=9 ("length (rest)")) -> (substring=w2735:string)
              n2259 = String Subset(string=w2724, offset (0)=25, length (rest)=9 ("length (rest)")) -> (substring=w2729:string)
              n2260 = String Subset(string=w2724, offset (0)=45, length (rest)=9 ("length (rest)")) -> (substring=w2737:string)
              n2261 = String Subset(string=w2724, offset (0)=0, length (rest)=14 ("length (rest)")) -> (substring=w2752:string)
              n2262 = String Subset(string=w2724, offset (0)=15, length (rest)=9 ("length (rest)")) -> (substring=w2755:string)
              n2263 = String Subset(string=w2724, offset (0)=65, length (rest)=9 ("length (rest)")) -> (substring=w2741:string)
              n2264 = Fract/Exp String To Number(string=w2727) -> (number=w2723:dbl)  [unwired: 3 in, 1 out]
              n2265 = Fract/Exp String To Number(string=w2749) -> (number=w2747:dbl)  [unwired: 3 in, 1 out]
              n2266 = Fract/Exp String To Number(string=w2735) -> (number=w2732:dbl)  [unwired: 3 in, 1 out]
              n2267 = Fract/Exp String To Number(string=w2729) -> (number=w2728:dbl)  [unwired: 3 in, 1 out]
              n2268 = Fract/Exp String To Number(string=w2737) -> (number=w2736:dbl)  [unwired: 3 in, 1 out]
              n2269 = Fract/Exp String To Number(string=w2752) -> (number=w2748:dbl)  [unwired: 3 in, 1 out]
              n2270 = Fract/Exp String To Number(string=w2755) -> (number=w2746:dbl)  [unwired: 3 in, 1 out]
              n2271 = Fract/Exp String To Number(string=w2741) -> (number=w2744:dbl)  [unwired: 3 in, 1 out]
              n2272 = Add(x=w2744, y=0.0) -> (x+y=w2740:dbl)
            }
            n2273 = for {
              N: w2632 -> [_]
              tunnel: w2639 -> [w2687]
              tunnel: w2638 -> [w2686]
              tunnel: [w2676] -> w2592 mode=indexing
              tunnel: [w2675] -> w2585 mode=indexing
              tunnel: w2629 -> [_]
              tunnel: [w2664] -> w2590 mode=indexing
              tunnel: [w2669] -> w2587 mode=indexing
              tunnel: [w2665] -> w2577 mode=indexing
              tunnel: [w2660] -> w2552 mode=indexing
              tunnel: [w2656] -> w2533 mode=indexing
              tunnel: [w2651] -> w2493 mode=indexing
              (unwired) 1.0 ("x")
              (unwired) TRUE ("line mode (F)")
              n2274 = Read from Text File "Read File"(file (use dialog)=w2687, error in=w2686) -> (text=w2652:string)  [unwired: 2 in, 3 out]
              n2275 = local write "String 12"(w2652) -> ()
              n2276 = String Subset(string=w2652, offset (0)=85, length (rest)=9 ("length (rest)")) -> (substring=w2654:string)
              n2277 = String Subset(string=w2652, offset (0)=35, length (rest)=9 ("length (rest)")) -> (substring=w2677:string)
              n2278 = String Subset(string=w2652, offset (0)=55, length (rest)=9 ("length (rest)")) -> (substring=w2662:string)
              n2279 = String Subset(string=w2652, offset (0)=25, length (rest)=9 ("length (rest)")) -> (substring=w2658:string)
              n2280 = String Subset(string=w2652, offset (0)=45, length (rest)=9 ("length (rest)")) -> (substring=w2667:string)
              n2281 = String Subset(string=w2652, offset (0)=15, length (rest)=9 ("length (rest)")) -> (substring=w2683:string)
              n2282 = String Subset(string=w2652, offset (0)=0, length (rest)=14 ("length (rest)")) -> (substring=w2680:string)
              n2283 = String Subset(string=w2652, offset (0)=65, length (rest)=9 ("length (rest)")) -> (substring=w2670:string)
              n2284 = Fract/Exp String To Number(string=w2654) -> (number=w2651:dbl)  [unwired: 3 in, 1 out]
              n2285 = Fract/Exp String To Number(string=w2677) -> (number=w2675:dbl)  [unwired: 3 in, 1 out]
              n2286 = Fract/Exp String To Number(string=w2662) -> (number=w2660:dbl)  [unwired: 3 in, 1 out]
              n2287 = Fract/Exp String To Number(string=w2658) -> (number=w2656:dbl)  [unwired: 3 in, 1 out]
              n2288 = Fract/Exp String To Number(string=w2667) -> (number=w2665:dbl)  [unwired: 3 in, 1 out]
              n2289 = Fract/Exp String To Number(string=w2683) -> (number=w2664:dbl)  [unwired: 3 in, 1 out]
              n2290 = Fract/Exp String To Number(string=w2680) -> (number=w2676:dbl)  [unwired: 3 in, 1 out]
              n2291 = Fract/Exp String To Number(string=w2670) -> (number=w2673:dbl)  [unwired: 3 in, 1 out]
              n2292 = Add(x=w2673, y=0.0) -> (x+y=w2669:dbl)
            }
            n2293 = Delete From Array(array=w2535, index=0) -> (array with subset deleted=w2508:dbl[])  [unwired: 1 in, 1 out]
            n2294 = Delete From Array(array=w2598, index=0) -> (array with subset deleted=w2571:dbl[])  [unwired: 1 in, 1 out]
            n2295 = Delete From Array(array=w2578, index=0) -> (array with subset deleted=w2566:dbl[])  [unwired: 1 in, 1 out]
            n2296 = Delete From Array(array=w2596, index=0) -> (array with subset deleted=w2597:dbl[])  [unwired: 1 in, 1 out]
            n2297 = call-poly <vilib>:"Mean.vi"("X"=w2508) -> ("mean"=→"КОФ2 4":dbl)  [unwired: 1 out]
            n2298 = call-poly <vilib>:"Mean.vi"("X"=w2571) -> ("mean"=→"КОФ3":dbl)  [unwired: 1 out]
            n2299 = call-poly <vilib>:"Mean.vi"("X"=w2566) -> ("mean"=→"CP3":dbl)  [unwired: 1 out]
            n2300 = Delete From Array(array=w2560, index=0) -> (array with subset deleted=w2487:dbl[])  [unwired: 1 in, 1 out]
            n2301 = Delete From Array(array=w2499, index=0) -> (array with subset deleted=w2486:dbl[])  [unwired: 1 in, 1 out]
            n2302 = Delete From Array(array=w2539, index=0) -> (array with subset deleted=w2510:dbl[])  [unwired: 1 in, 1 out]
            n2303 = Delete From Array(array=w2617, index=0) -> (array with subset deleted=w2572:dbl[])  [unwired: 1 in, 1 out]
            n2304 = Delete From Array(array=w2583, index=0) -> (array with subset deleted=w2568:dbl[])  [unwired: 1 in, 1 out]
            "array w/ subset deleted" <- w2568
            n2305 = Delete From Array(array=w2614, index=0) -> (array with subset deleted=w2615:dbl[])  [unwired: 1 in, 1 out]
            n2306 = call-poly <vilib>:"Mean.vi"("X"=w2510) -> ("mean"=→"КОФ2 2":dbl)  [unwired: 1 out]
            n2307 = call-poly <vilib>:"Mean.vi"("X"=w2572) -> ("mean"=→"КОФ1":dbl)  [unwired: 1 out]
            n2308 = Bundle "Bundle"(w2487, w2486) -> (w2492:cluster{dbl[], dbl[]})  [unwired: 1 in]
            n2309 = Bundle "Bundle"(w2487, w2615) -> (w2479:cluster{dbl[], dbl[]})  [unwired: 1 in]
            n2310 = Delete From Array(array=w2494, index=0) -> (array with subset deleted=w2482:dbl[])  [unwired: 1 in, 1 out]
            n2311 = Delete From Array(array=w2495, index=0) -> (array with subset deleted=w2484:dbl[])  [unwired: 1 in, 1 out]
            n2312 = Delete From Array(array=w2605, index=0) -> (array with subset deleted=w2606:dbl[])  [unwired: 1 in, 1 out]
            n2313 = Delete From Array(array=w2493, index=0) -> (array with subset deleted=w2480:dbl[])  [unwired: 1 in, 1 out]
            n2314 = Delete From Array(array=w2587, index=0) -> (array with subset deleted=w2588:dbl[])  [unwired: 1 in, 1 out]
            n2315 = Delete From Array(array=w2612, index=0) -> (array with subset deleted=w2518:dbl[])  [unwired: 1 in, 1 out]
            n2316 = Delete From Array(array=w2558, index=0) -> (array with subset deleted=w2514:dbl[])  [unwired: 1 in, 1 out]
            n2317 = Delete From Array(array=w2594, index=0) -> (array with subset deleted=w2516:dbl[])  [unwired: 1 in, 1 out]
            n2318 = Delete From Array(array=w2554, index=0) -> (array with subset deleted=w2512:dbl[])  [unwired: 1 in, 1 out]
            n2319 = Delete From Array(array=w2603, index=0) -> (array with subset deleted=w2517:dbl[])  [unwired: 1 in, 1 out]
            n2320 = Delete From Array(array=w2556, index=0) -> (array with subset deleted=w2513:dbl[])  [unwired: 1 in, 1 out]
            n2321 = Delete From Array(array=w2537, index=0) -> (array with subset deleted=w2509:dbl[])  [unwired: 1 in, 1 out]
            n2322 = Delete From Array(array=w2581, index=0) -> (array with subset deleted=w2567:dbl[])  [unwired: 1 in, 1 out]
            n2323 = Delete From Array(array=w2608, index=0) -> (array with subset deleted=w2569:dbl[])  [unwired: 1 in, 1 out]
            n2324 = Delete From Array(array=w2585, index=0) -> (array with subset deleted=w2515:dbl[])  [unwired: 1 in, 1 out]
            n2325 = Delete From Array(array=w2552, index=0) -> (array with subset deleted=w2511:dbl[])  [unwired: 1 in, 1 out]
            n2326 = Delete From Array(array=w2533, index=0) -> (array with subset deleted=w2507:dbl[])  [unwired: 1 in, 1 out]
            n2327 = Delete From Array(array=w2577, index=0) -> (array with subset deleted=w2565:dbl[])  [unwired: 1 in, 1 out]
            n2328 = Delete From Array(array=w2590, index=0) -> (array with subset deleted=w2570:dbl[])  [unwired: 1 in, 1 out]
            n2329 = Delete From Array(array=w2600, index=0) -> (array with subset deleted=w2483:dbl[])  [unwired: 1 in, 1 out]
            n2330 = Delete From Array(array=w2610, index=0) -> (array with subset deleted=w2485:dbl[])  [unwired: 1 in, 1 out]
            n2331 = Delete From Array(array=w2592, index=0) -> (array with subset deleted=w2481:dbl[])  [unwired: 1 in, 1 out]
            n2332 = Bundle "Bundle"(w2487, w2518) -> (w2505:cluster{dbl[], dbl[]})  [unwired: 1 in]
            n2333 = Bundle "Bundle"(w2487, w2572) -> (w2506:cluster{dbl[], dbl[]})  [unwired: 1 in]
            n2334 = Bundle "Bundle"(w2518, w2514) -> (w2520:cluster{dbl[], dbl[]})  [unwired: 1 in]
            n2335 = Bundle "Bundle"(w2483, w2482) -> (w2490:cluster{dbl[], dbl[]})  [unwired: 1 in]
            n2336 = Bundle "Bundle"(w2516, w2512) -> (w2522:cluster{dbl[], dbl[]})  [unwired: 1 in]
            n2337 = Bundle "Bundle"(w2483, w2516) -> (w2626:cluster{dbl[], dbl[]})  [unwired: 1 in]
            n2338 = Bundle "Bundle"(w2483, w2512) -> (w2550:cluster{dbl[], dbl[]})  [unwired: 1 in]
            n2339 = Bundle "Bundle"(w2483, w2571) -> (w2636:cluster{dbl[], dbl[]})  [unwired: 1 in]
            n2340 = Bundle "Bundle"(w2483, w2566) -> (w2574:cluster{dbl[], dbl[]})  [unwired: 1 in]
            n2341 = Bundle "Bundle"(w2483, w2597) -> (w2621:cluster{dbl[], dbl[]})  [unwired: 1 in]
            n2342 = Bundle "Bundle"(w2517, w2513) -> (w2521:cluster{dbl[], dbl[]})  [unwired: 1 in]
            n2343 = Bundle "Bundle"(w2485, w2484) -> (w2491:cluster{dbl[], dbl[]})  [unwired: 1 in]
            n2344 = Bundle "Bundle"(w2485, w2517) -> (w2628:cluster{dbl[], dbl[]})  [unwired: 1 in]
            n2345 = Bundle "Bundle"(w2485, w2513) -> (w2551:cluster{dbl[], dbl[]})  [unwired: 1 in]
            n2346 = Bundle "Bundle"(w2485, w2567) -> (w2575:cluster{dbl[], dbl[]})  [unwired: 1 in]
            n2347 = Bundle "Bundle"(w2485, w2569) -> (w2637:cluster{dbl[], dbl[]})  [unwired: 1 in]
            n2348 = Bundle "Bundle"(w2485, w2606) -> (w2619:cluster{dbl[], dbl[]})  [unwired: 1 in]
            n2349 = Bundle "Bundle"(w2515, w2511) -> (w2523:cluster{dbl[], dbl[]})  [unwired: 1 in]
            n2350 = Bundle "Bundle"(w2481, w2480) -> (w2489:cluster{dbl[], dbl[]})  [unwired: 1 in]
            n2351 = Bundle "Bundle"(w2481, w2515) -> (w2627:cluster{dbl[], dbl[]})  [unwired: 1 in]
            n2352 = Bundle "Bundle"(w2481, w2511) -> (w2549:cluster{dbl[], dbl[]})  [unwired: 1 in]
            n2353 = Bundle "Bundle"(w2481, w2565) -> (w2573:cluster{dbl[], dbl[]})  [unwired: 1 in]
            n2354 = Bundle "Bundle"(w2481, w2570) -> (w2635:cluster{dbl[], dbl[]})  [unwired: 1 in]
            n2355 = Bundle "Bundle"(w2481, w2588) -> (w2620:cluster{dbl[], dbl[]})  [unwired: 1 in]
            n2356 = call-poly <vilib>:"Mean.vi"("X"=w2568) -> ("mean"=→"CP1":dbl)  [unwired: 1 out]
            n2357 = call-poly <vilib>:"Mean.vi"("X"=w2509) -> ("mean"=→"КОФ2 3":dbl)  [unwired: 1 out]
            n2358 = call-poly <vilib>:"Mean.vi"("X"=w2567) -> ("mean"=→"CP2":dbl)  [unwired: 1 out]
            n2359 = call-poly <vilib>:"Mean.vi"("X"=w2569) -> ("mean"=→"КОФ2":dbl)  [unwired: 1 out]
            n2360 = call-poly <vilib>:"Mean.vi"("X"=w2507) -> ("mean"=→"КОФ2 5":dbl)  [unwired: 1 out]
            n2361 = call-poly <vilib>:"Mean.vi"("X"=w2565) -> ("mean"=→"CP4":dbl)  [unwired: 1 out]
            n2362 = call-poly <vilib>:"Mean.vi"("X"=w2570) -> ("mean"=→"КОФ4":dbl)  [unwired: 1 out]
            n2363 = Bundle "Bundle"(w2487, w2514) -> (w2478:cluster{dbl[], dbl[]})  [unwired: 1 in]
            n2364 = Bundle "Bundle"(w2487, w2568) -> (w2501:cluster{dbl[], dbl[]})  [unwired: 1 in]
            n2365 = Build Array "Build Array"(w2478, w2501) -> (w2504:cluster{dbl[], dbl[]}[])
            "XY Graph 17" <- w2504
            n2366 = Build Array "Build Array"(w2492, w2491, w2490, w2489) -> (→"Frequency ( Hz )":cluster{dbl[], dbl[]}[])
            n2367 = Build Array "Build Array"(w2520, w2521, w2522, w2523) -> (→"Air Temp ( °C ) vs Humidity ( % RH )":cluster{dbl[], dbl[]}[])
            n2368 = Build Array "Build Array"(w2505, w2628, w2626, w2627) -> (→"Air Temperature  ( °C )":cluster{dbl[], dbl[]}[])
            n2369 = Build Array "Build Array"(w2478, w2551, w2550, w2549) -> (→"Humidity ( %RH )":cluster{dbl[], dbl[]}[])
            n2370 = Build Array "Build Array"(w2506, w2637, w2636, w2635) -> (→"Coefficient Of Friction":cluster{dbl[], dbl[]}[])
            n2371 = Build Array "Build Array"(w2501, w2575, w2574, w2573) -> (→"Sample Temperature ( °C )":cluster{dbl[], dbl[]}[])
            n2372 = Build Array "Build Array"(w2479, w2619, w2621, w2620) -> (→"XY Graph 13":cluster{dbl[], dbl[]}[])
            n2373 = Bundle "Bundle"(w2487, w2510) -> (w2532:cluster{dbl[], dbl[]})  [unwired: 1 in]
            n2374 = Bundle "Bundle"(w2483, w2508) -> (w2530:cluster{dbl[], dbl[]})  [unwired: 1 in]
            n2375 = Bundle "Bundle"(w2485, w2509) -> (w2531:cluster{dbl[], dbl[]})  [unwired: 1 in]
            n2376 = Bundle "Bundle"(w2481, w2507) -> (w2529:cluster{dbl[], dbl[]})  [unwired: 1 in]
            n2377 = Build Array "Build Array"(w2532, w2531, w2530, w2529) -> (→"Stroke ( mm )":cluster{dbl[], dbl[]}[])
            n2378 = local write "XY Graph 16"(w2504) -> ()
          }
          frame #2 {
          }
          frame #3 {
            n2379 = local write "Numeric 8"(0 ("Numeric 8")) -> ()
            n2380 = local write "Numeric 11"(0 ("Numeric 11")) -> ()
            n2381 = local write "Numeric 12"(0 ("Numeric 12")) -> ()
            n2382 = local write "Numeric 13"(0 ("Numeric 13")) -> ()
            n2383 = property on="OPEN" class="Bool (strict)"("Visible"=TRUE) -> ()  [unwired: 2 in, 2 out]
            n2384 = local read "String Control 2"() -> (w2804:string)
            n2385 = local read "String Control 4"() -> (w2803:string)
            n2386 = local read "String Control 6"() -> (w2802:string)
            n2387 = local read "String Control 8"() -> (w2801:string)
            n2388 = Match Pattern(string=w2804, regular expression="Samples / cycle :- ") -> (after substring=w2818:string)  [unwired: 1 in, 3 out]
            n2389 = Match Pattern(string=w2804, regular expression="Frequency :- ") -> (after substring=w2837:string)  [unwired: 1 in, 3 out]
            n2390 = Match Pattern(string=w2803, regular expression="Samples / cycle :- ") -> (after substring=w2814:string)  [unwired: 1 in, 3 out]
            n2391 = Match Pattern(string=w2803, regular expression="Frequency :- ") -> (after substring=w2832:string)  [unwired: 1 in, 3 out]
            n2392 = Match Pattern(string=w2802, regular expression="Samples / cycle :- ") -> (after substring=w2810:string)  [unwired: 1 in, 3 out]
            n2393 = Match Pattern(string=w2802, regular expression="Frequency :- ") -> (after substring=w2827:string)  [unwired: 1 in, 3 out]
            n2394 = Match Pattern(string=w2801, regular expression="Samples / cycle :- ") -> (after substring=w2806:string)  [unwired: 1 in, 3 out]
            n2395 = Match Pattern(string=w2801, regular expression="Frequency :- ") -> (after substring=w2822:string)  [unwired: 1 in, 3 out]
            n2396 = String Subset(string=w2818, length (rest)=6 ("length (rest)")) -> (substring=w2820:string)  [unwired: 1 in]
            n2397 = String Subset(string=w2837, length (rest)=9 ("length (rest)")) -> (substring=w2839:string)  [unwired: 1 in]
            n2398 = String Subset(string=w2814, length (rest)=6 ("length (rest)")) -> (substring=w2816:string)  [unwired: 1 in]
            n2399 = String Subset(string=w2832, length (rest)=9 ("length (rest)")) -> (substring=w2834:string)  [unwired: 1 in]
            n2400 = String Subset(string=w2810, length (rest)=6 ("length (rest)")) -> (substring=w2812:string)  [unwired: 1 in]
            n2401 = String Subset(string=w2827, length (rest)=9 ("length (rest)")) -> (substring=w2829:string)  [unwired: 1 in]
            n2402 = String Subset(string=w2806, length (rest)=6 ("length (rest)")) -> (substring=w2808:string)  [unwired: 1 in]
            n2403 = String Subset(string=w2822, length (rest)=9 ("length (rest)")) -> (substring=w2824:string)  [unwired: 1 in]
            n2404 = Fract/Exp String To Number(string=w2820) -> (number=w2800:dbl)  [unwired: 3 in, 1 out]
            n2405 = Fract/Exp String To Number(string=w2839) -> (number=w2840:dbl)  [unwired: 3 in, 1 out]
            n2406 = Fract/Exp String To Number(string=w2816) -> (number=w2799:dbl)  [unwired: 3 in, 1 out]
            n2407 = Fract/Exp String To Number(string=w2834) -> (number=w2835:dbl)  [unwired: 3 in, 1 out]
            n2408 = Fract/Exp String To Number(string=w2812) -> (number=w2798:dbl)  [unwired: 3 in, 1 out]
            n2409 = Fract/Exp String To Number(string=w2829) -> (number=w2830:dbl)  [unwired: 3 in, 1 out]
            n2410 = Fract/Exp String To Number(string=w2808) -> (number=w2797:dbl)  [unwired: 3 in, 1 out]
            n2411 = Fract/Exp String To Number(string=w2824) -> (number=w2825:dbl)  [unwired: 3 in, 1 out]
            n2412 = local write "sample1"(w2800) -> ()
            n2413 = local write "freq1"(w2840) -> ()
            n2414 = local write "sample2"(w2799) -> ()
            n2415 = local write "freq2"(w2835) -> ()
            n2416 = local write "sample3"(w2798) -> ()
            n2417 = local write "freq3"(w2830) -> ()
            n2418 = local write "sample4"(w2797) -> ()
            n2419 = local write "freq 4"(w2825) -> ()
          }
        }
      }
    }
    n2420 = case shown="True" w2398 {
      selector: w2398 -> [_ w2417]
      frame False {
      }
      frame True {
        n2421 = Not(x=w2417) -> (.not. x?=w2413:bool)
        n2422 = local write "service 3"(w2413) -> ()
        n2423 = local write "OPEN 6"(w2413) -> ()
        n2424 = call <vilib>:"System Exec.vi"("wait until completion? (T)"=TRUE, "command line"="C:\\LAB-IQ\\Scar View.exe") -> ("error out"=→"error out 5":errorcluster)  [unwired: 6 in, 3 out]
      }
    }
    n2425 = case shown="\"Acquire\", Default" w2407 {
      frame "Acquire", Default {
        # "Elapsed time\ncof\nstroke\nAir temp\nTemp\nHumidity"
        n2426 = disable-structure shown="Disabled" {
          frame Disabled {
            n2427 = local read "Flag"() -> (w3116:dbl)
            n2428 = local read "RUN"() -> (w3113:bool)
            n2429 = Not(x=w3113) -> (.not. x?=w3112:bool)
            n2430 = Equal?(x=w3116, y=10.0) -> (x = y?=w3114:bool)
            n2431 = And(x=w3114, y=w3112) -> (x .and. y?=w3111:bool)
            n2432 = case shown="True" w3111 {
              frame False {
              }
              frame True {
                w3117 = FALSE ("Heater Button")
                n2433 = local write "Humidity"(w3117) -> ()
                n2434 = local write "Heater Button"(w3117) -> ()
              }
            }
          }
          frame Enabled {
          }
        }
        n2435 = disable-structure shown="Disabled" {
          frame Disabled {
            n2436 = case shown="True" {
              selector: _ -> [_ _]
              frame False {
              }
              frame True {
                w3162 = TRUE ("Heater")
                n2437 = local write "Humidity"(w3162) -> ()
                n2438 = local write "Heater Button"(w3162) -> ()
                n2439 = local read "TEST STANDARD"() -> (w3165:T5)
